vi "Write_userEventInstanceCmd.vi"(8 "error in (no error)":errorcluster, 10 "userEventInstanceCmd":T1, 11 "TcpServerCmd in":refnum<class "TcpServerCmd.lvclass">) -> (0 "error out":errorcluster, 3 "TcpServerCmd out":refnum<class "TcpServerCmd.lvclass">)   [LabVIEW 2018, in "TcpServerCmd.lvclass"]
doc: "Write UserEvent cluster, with user event instances inside."
uses:
  TcpServerCmd.lvclass
  typedef/userEventTypeDef.ctl
  TcpServerBase/typedef/tcpPacketTypeDef.ctl
  typedef/ackTypeDef.ctl
  typedef/eventTypeDef.ctl
  TcpServerCmd.lvclass/TcpServerCmd.ctl
  TcpServerBase/TcpServerBase.lvclass
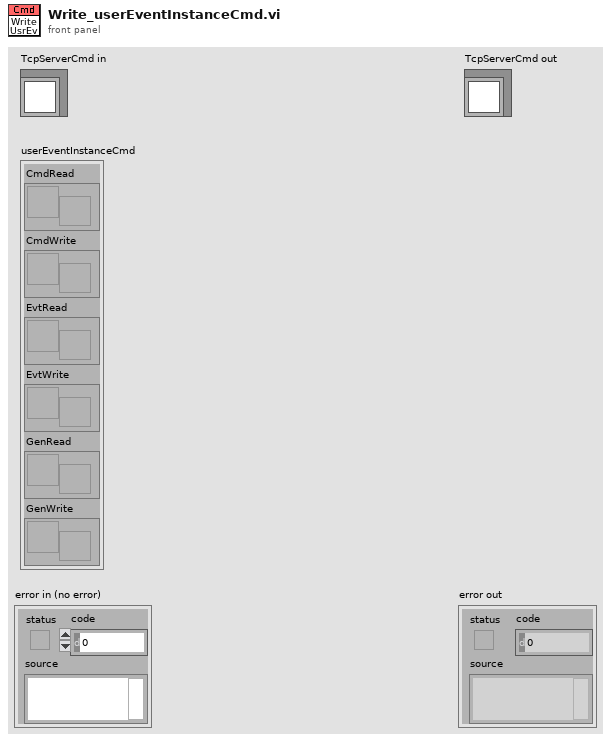
[diagram p1: front panel]
types:
  T1 = typedef "TcpServerCmd.lvclass/userEventTypeDef.ctl" = cluster{"CmdRead":refnum<user-event>, "CmdWrite":refnum<user-event>, "EvtRead":refnum<user-event>, "EvtWrite":refnum<user-event>, "GenRead":refnum<user-event>, "GenWrite":refnum<user-event>}
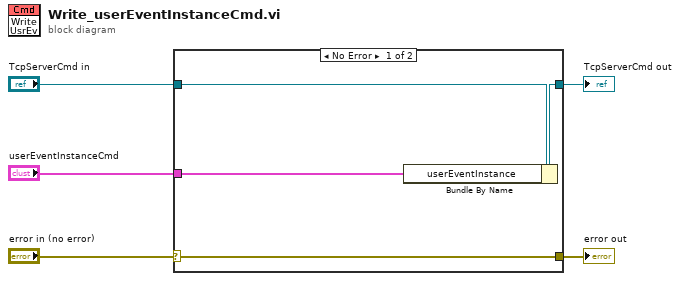
[diagram p0: block diagram]
diagram:
  n1 = case shown="No Error" "error in (no error)" {
    selector: "error in (no error)" -> [w9 w10]
    tunnel: [w9 w10] -> w4
    tunnel: [w7 w11] -> w2
    tunnel: "TcpServerCmd in" -> [w8 w11]
    tunnel: "userEventInstanceCmd" -> [w6 _]
    frame No Error {
      n2 = Bundle By Name(cluster=w8, "userEventInstance"=w6) -> (w7:refnum<class "TcpServerCmd.lvclass">)
    }
    frame Error {
    }
  }
  "error out" <- w4
  "TcpServerCmd out" <- w2
